vi "Read Valve Capillary Line.vi"(11 "Capillary Line in":refnum<class "Capillary Line.lvclass">) -> (2 "Actor Framework:Message Enqueuer":refnum<class "Message Enqueuer.lvclass">, 3 "Capillary Line out":refnum<class "Capillary Line.lvclass">)   [LabVIEW 2015, in "cRIO-Carbondioxide.lvlib" / "CO2-Actor.lvlib" / "Capillary Line.lvclass"]
uses:
  Capillary Line.lvclass
  <vilib>/ActorFramework/Message Enqueuer/Message Enqueuer.lvclass
  Capillary Line.lvclass/Capillary Line.ctl
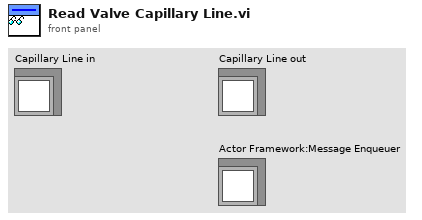
[diagram p1: front panel]
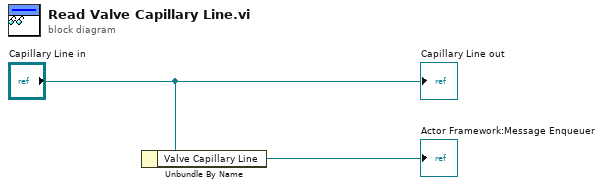
[diagram p0: block diagram]
diagram:
  n1 = Unbundle By Name("Capillary Line in") -> ("Valve Capillary Line"=→"Actor Framework:Message Enqueuer":refnum<class "Message Enqueuer.lvclass">)
  "Capillary Line out" <- "Capillary Line in"
